vi "config select and copy.vi"(8 "error in (no error)":errorcluster, 11 "Config in":path) -> (0 "error out":errorcluster, 3 "UUT Path":path, 5 "Current Configuration":string)   [LabVIEW 2011]
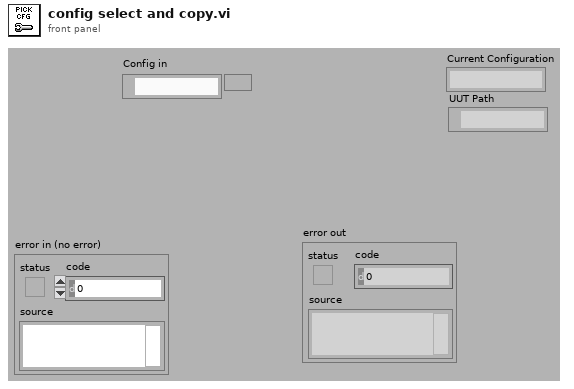
[diagram p1: front panel]
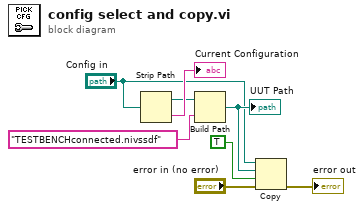
[diagram p0: block diagram]
diagram:
  n1 = Strip Path(path="Config in") -> (stripped path=w2:path, name=→"Current Configuration":string)
  n2 = Build Path(base path=w2, name or relative path="TESTBENCHconnected.nivssdf") -> (appended path=w6:path)
  "UUT Path" <- w6
  n3 = Copy(8:"error in (no error)", 9:TRUE ("overwrite (F)"), 10:w6, 11:"Config in") -> (0:→"error out":errorcluster)  [unwired: 1 in, 2 out]
